vi "Rotation stage shgv6.vi"() -> ()   [LabVIEW 2020]
doc: "Shows how to move a motor to an absolute position."
uses:
  <vilib>/Utility/error.llb/DialogType.ctl
  <vilib>/DAQmx/read.llb/DAQmx Read (Analog 1D Wfm NChan 1Samp).vi
  <vilib>/DAQmx/read.llb/DAQmx Read (Counter 1D U32 1Chan NSamp).vi
  <vilib>/DAQmx/create/channels.llb/DAQmx Create Channel (CI-Period).vi
  <vilib>/DAQmx/create/channels.llb/DAQmx Create Channel (CO-Pulse Generation-Frequency).vi
  <vilib>/DAQmx/configure/timing.llb/DAQmx Timing (Implicit).vi
  <vilib>/DAQmx/miscellaneous.llb/DAQmx Fill In Error Info.vi
  <vilib>/DAQmx/create/channels.llb/DAQmx Create Channel (AI-Current-Basic).vi
  <vilib>/DAQmx/configure/timing.llb/DAQmx Timing (Sample Clock).vi
  <resource>/objmgr/daqmx.rc
panel:
  in  "stop":bool
  in  "MG17Motor":refnum<k7>(container)
  in  "Home":bool
  in  "Move Relative":bool
  in  "Rel Move Size":dbl=1.0 min=-10.0 max=10.0 format="%.2f"
  in  "Set Rel Move Size":bool
  in  "Stop":bool
  out "Actual Sample Rate":dbl=1000.0 format="%0.2f"
  out "Reference Channel":waveform(dbl)[](graph)
  out "Consumer Iteration 3":i32=1109257
  out "Producer Iteration 3":i32=1109256
  out "error out 3":errorcluster
  out "Loop Time (ms) 3":u32=10
  in  "Duty Cycle":dbl=0.5 format="%.6f"
  out "Input.BufSize":u32=1000000 format="%.0p"
  out "PC-PMT":u32[](graph)
  out "Consumer Iteration 2":i32=1109257
  in  "number of samples per channel 2":i32=5000
  out "Producer Iteration 2":i32=1109256
  out "error out 2":errorcluster
  out "Loop Time (ms) 2":u32=10
  in  "dwell time (ms)":dbl=1.0 format="%.6f"
  in  "Photon Input (PFI)":tag="/Dev1/PFI0"
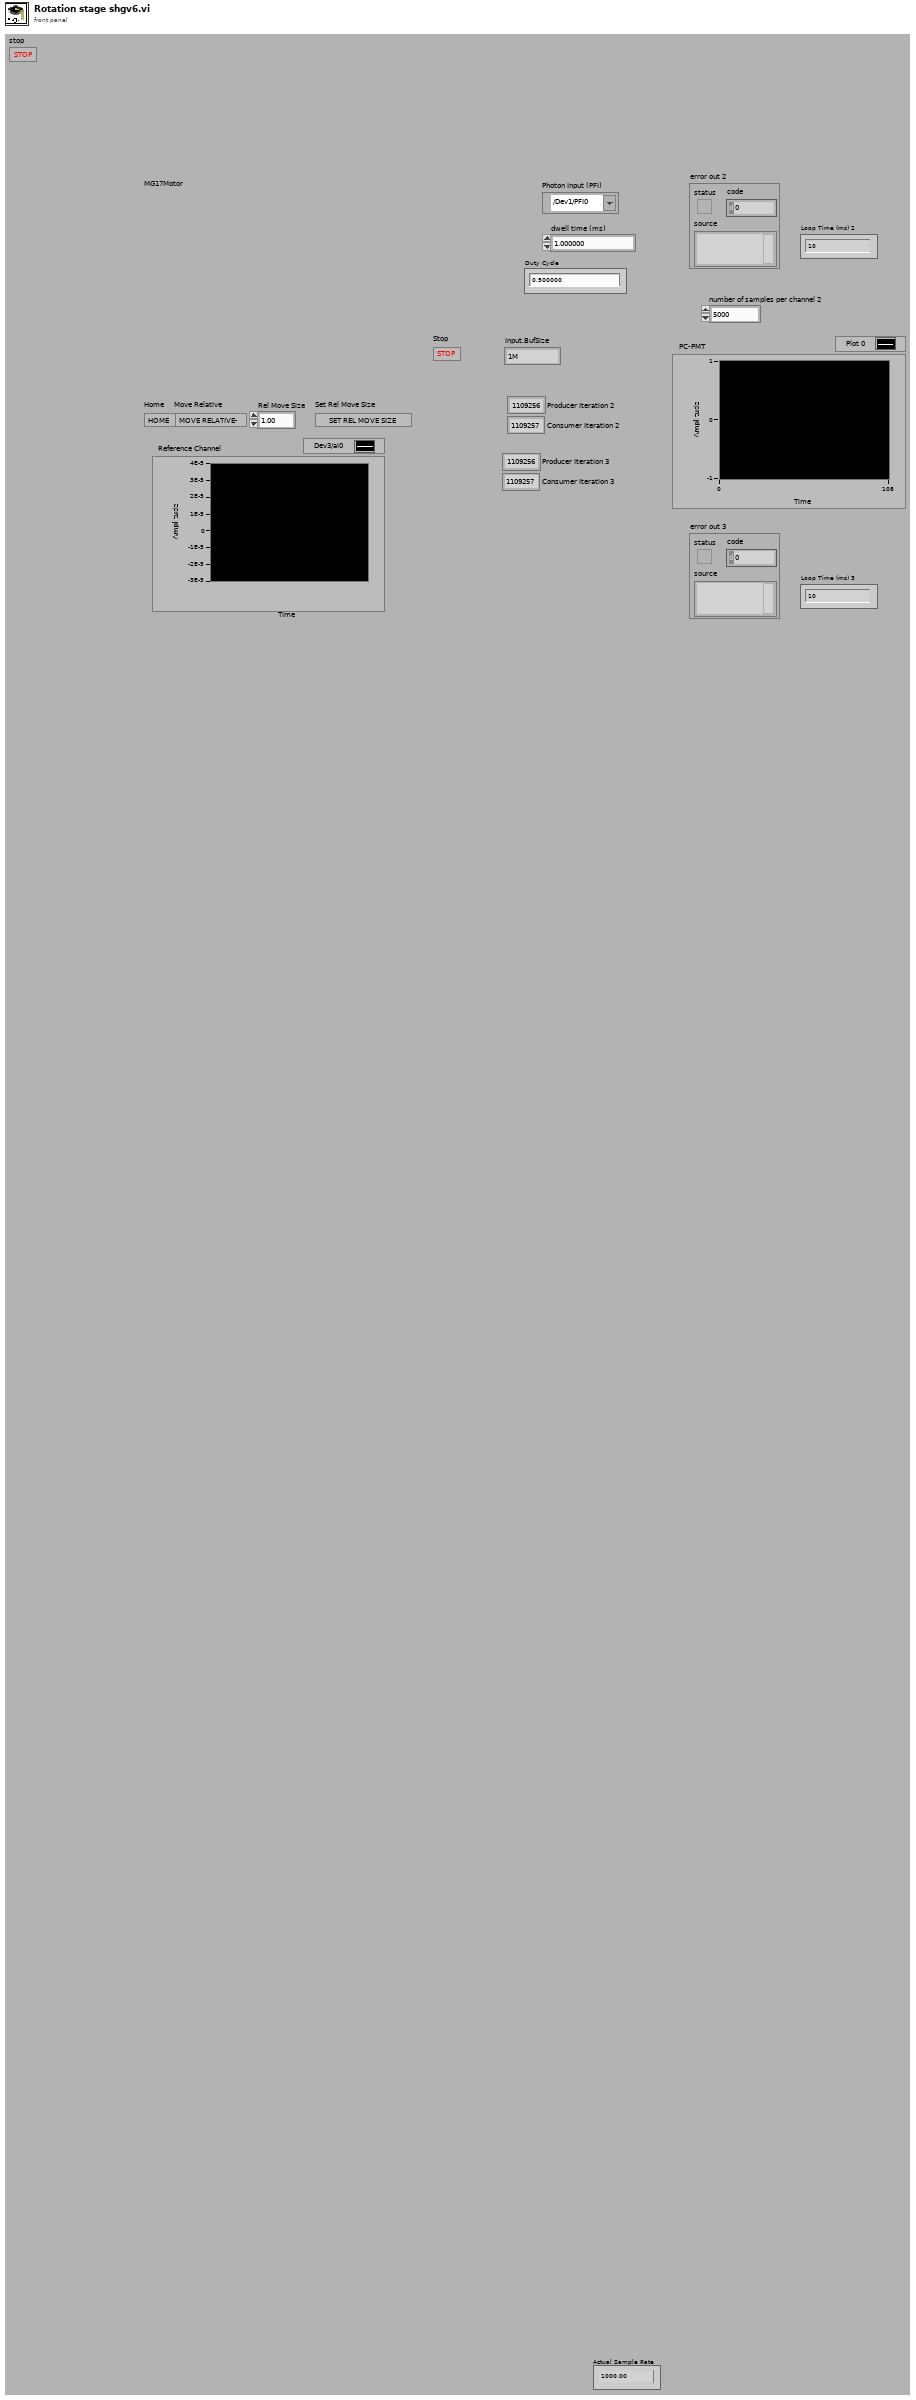
[diagram p1: front panel]
types:
  T1 = enum16{"open", "open or create", "create or replace", "create", "open (read-only)"}
  T2 = typedef "DialogType.ctl" = u16
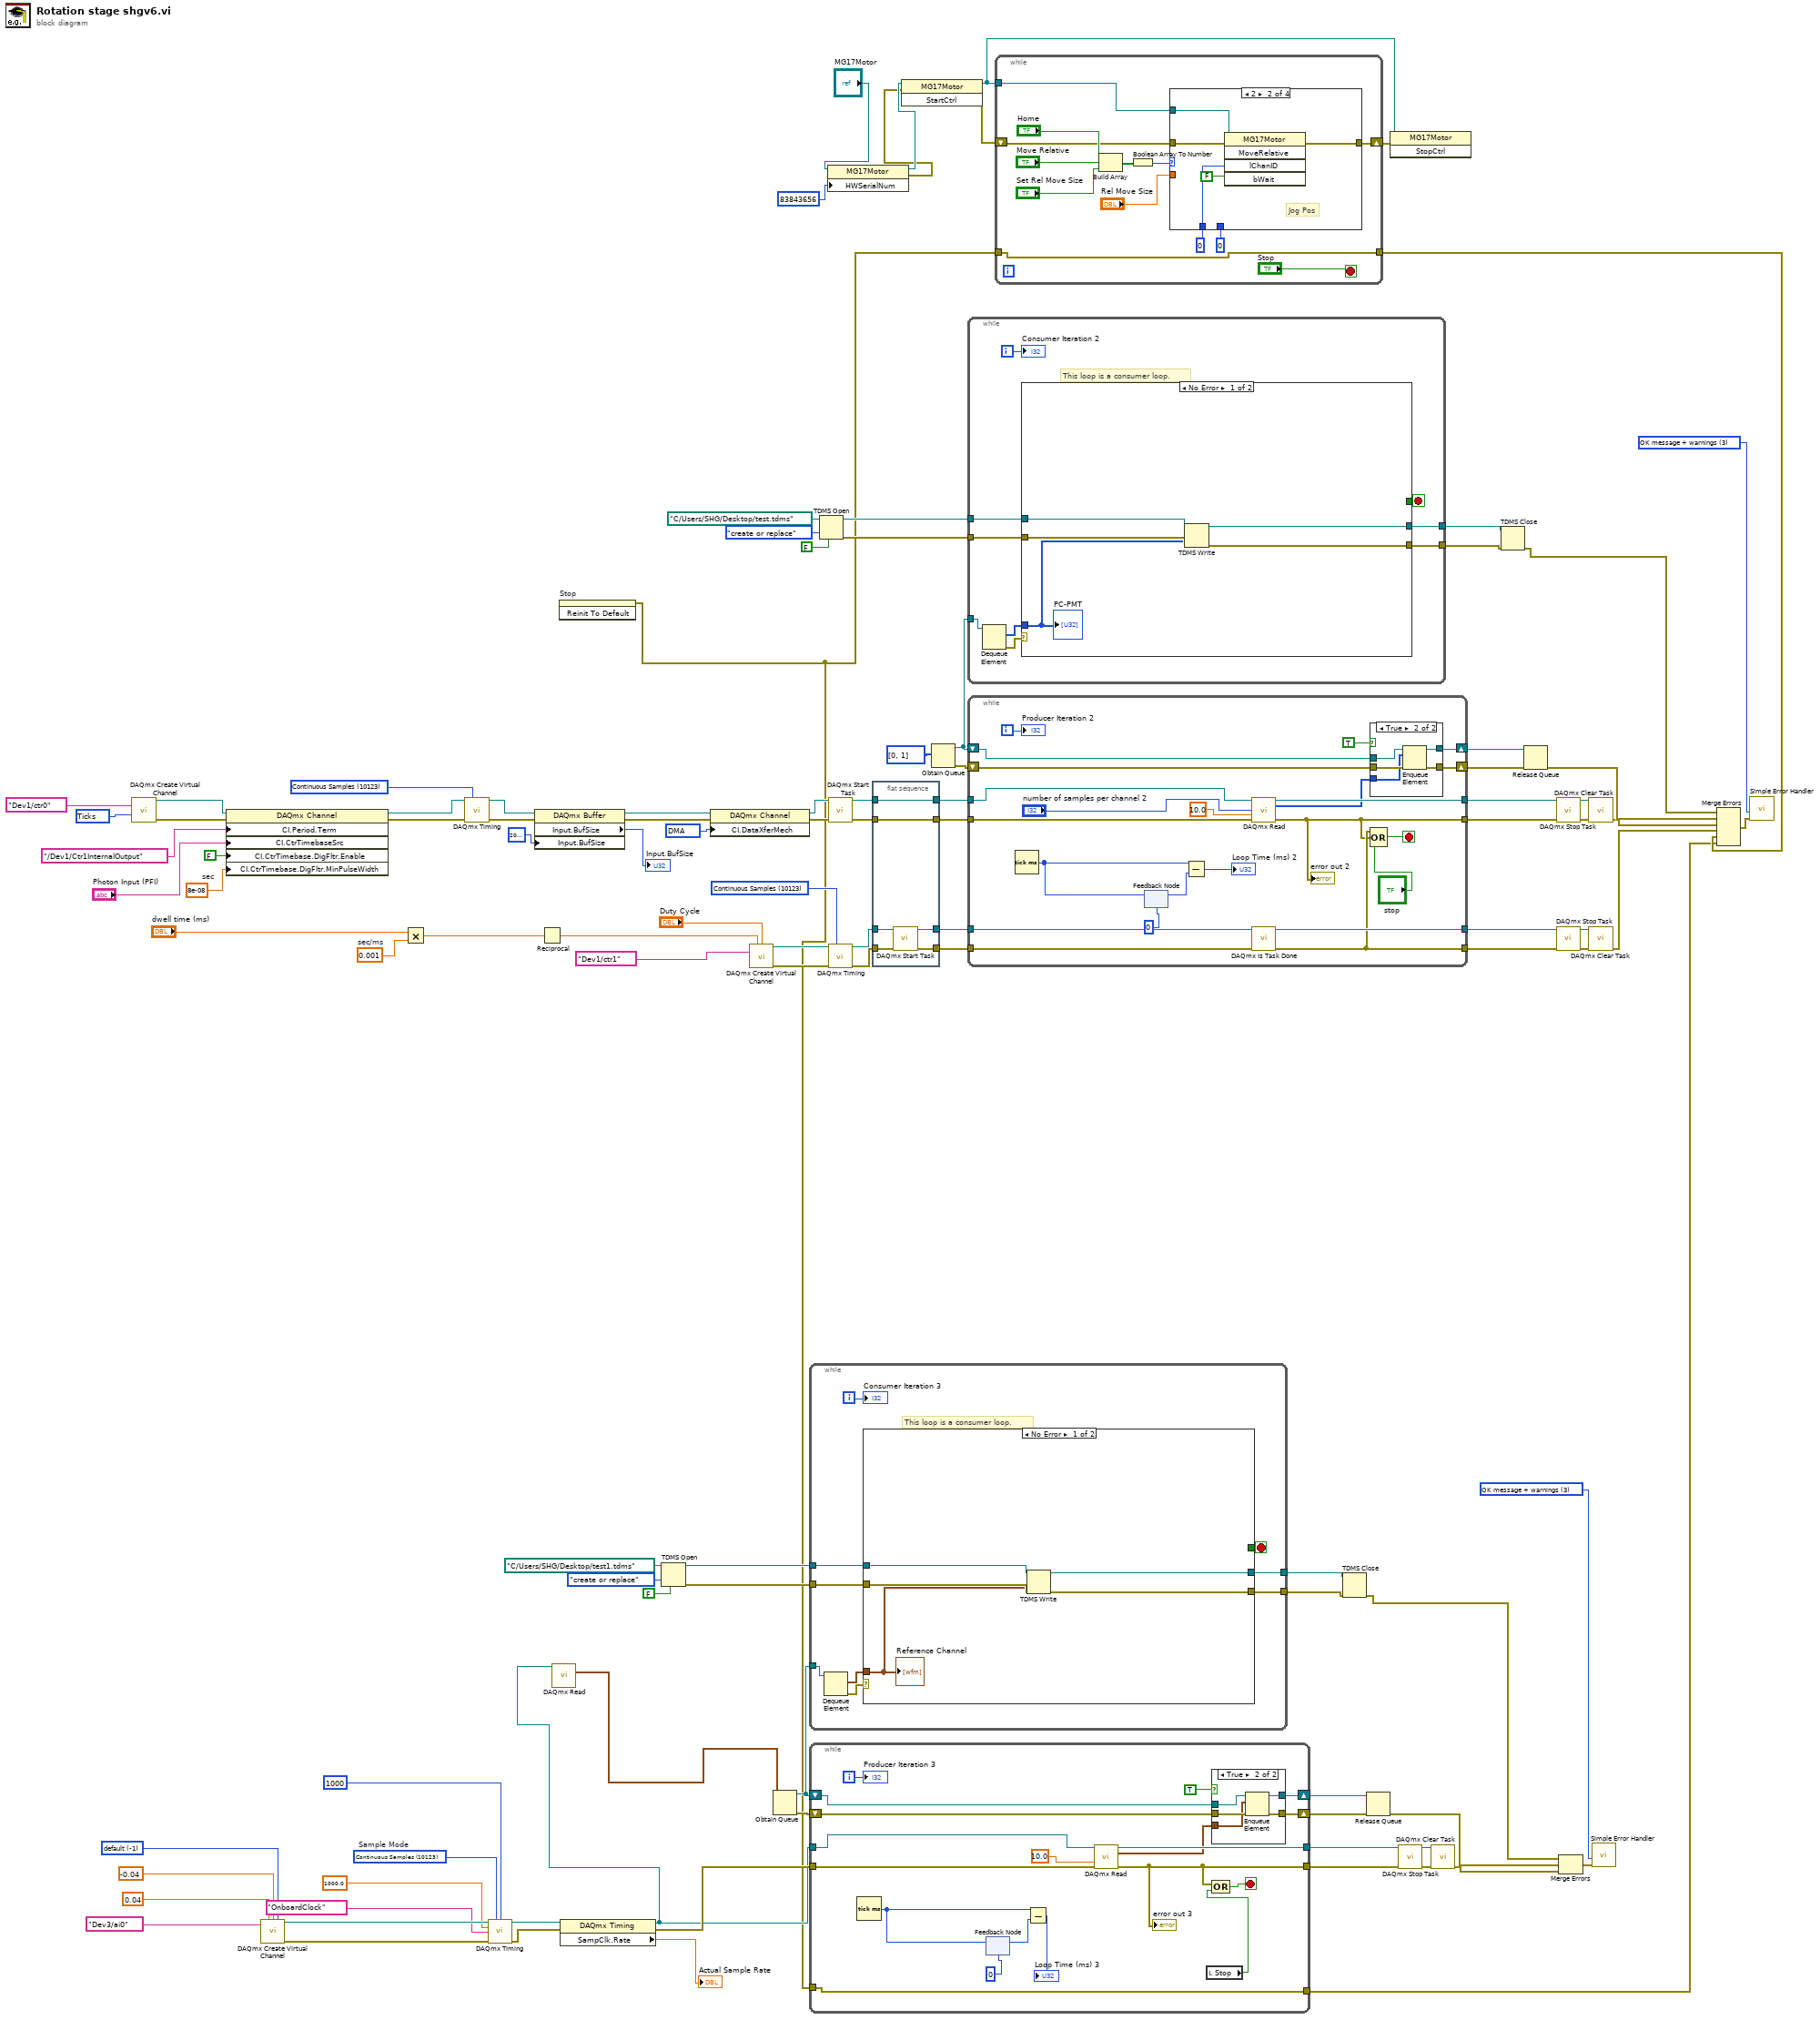
[diagram p0: block diagram]
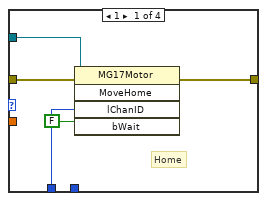
[diagram p2: hidden frame]
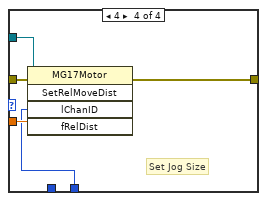
[diagram p4: hidden frame]
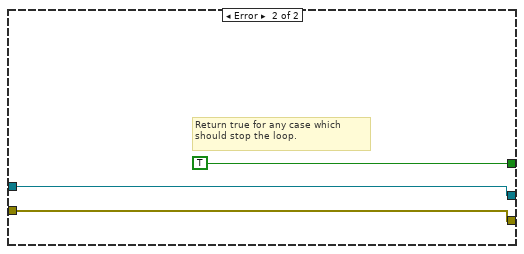
[diagram p5: hidden frame]
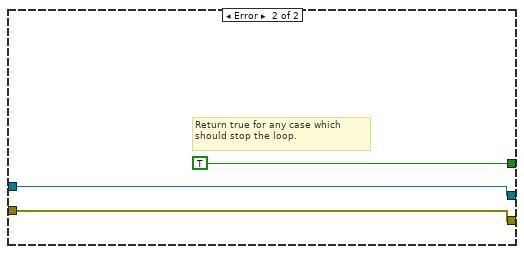
[diagram p7: hidden frame]
diagram:
  w16 = -1 items=["default"=-1, "RSE"=10083, "NRSE"=10078, "Differential"=10106, "Pseudodifferential"=12529] ("Terminal Configuration")
  w24 = 10123 items=["Finite Samples"=10178, "Continuous Samples"=10123, "Hardware Timed Single Point"=12522]  # Sample Mode
  w34 = T2 3 items=["no dialog", "OK message", "continue or stop message", "OK message + warnings", "continue/stop + warnings"] ("type of dialog (OK msg:1)")
  w55 = T2 3 items=["no dialog", "OK message", "continue or stop message", "OK message + warnings", "continue/stop + warnings"] ("type of dialog (OK msg:1)")
  w60 = 8e-08  # sec
  w71 = 10054 items=["DMA"=10054, "Interrupts"=10204, "Programmed I/O"=10264, "USB Bulk"=12590] ("CI.DataXferMech")
  w91 = 0.001  # sec/ms
  w101 = 10304 items=["Seconds"=10364, "Ticks"=10304, "From Custom Scale"=10065] ("units")
  w102 = 10123 items=["Finite Samples"=10178, "Continuous Samples"=10123, "Hardware Timed Single Point"=12522] ("sample mode")
  w103 = 10123 items=["Finite Samples"=10178, "Continuous Samples"=10123, "Hardware Timed Single Point"=12522] ("sample mode")
  n1 = call-poly <vilib>:"DAQmx Create Virtual Channel.vi"("counter"=tag "Dev1/ctr0", "units"=w101) -> ("task out"=w98:refnum<k21>, "error out"=w97:errorcluster)  [unwired: 12 in]
  n2 = property class="DAQmx Channel"(reference=w98, error in=w97, "CI.Period.Term"=tag "/Dev1/Ctr1InternalOutput", "CI.CtrTimebaseSrc"="Photon Input (PFI)", "CI.CtrTimebase.DigFltr.Enable"=FALSE, "CI.CtrTimebase.DigFltr.MinPulseWidth"=w60) -> (reference out=w96:refnum<k21>, error out=w95:errorcluster)
  n3 = call-poly <vilib>:"DAQmx Create Virtual Channel.vi"("maximum value"=0.04 ("Max Voltage"), "minimum value"=-0.04 ("Min Voltage"), "input terminal configuration"=w16, "physical channels"=tag "Dev3/ai0" ("Physical Channel")) -> ("task out"=w22:refnum<k21>, "error out"=w23:errorcluster)  [unwired: 10 in]
  n4 = Multiply(x="dwell time (ms)", y=w91) -> (x*y=w90:dbl)
  n5 = call-poly <vilib>:"DAQmx Timing.vi"("task/channels in"=w96, "sample mode"=w102, "error in"=w95) -> ("task out"=w66:refnum<k21>, "error out"=w65:errorcluster)  [unwired: 11 in]
  n6 = call-poly <vilib>:"DAQmx Timing.vi"("task/channels in"=w22, "sample mode"=w24, "samples per channel"=1000 ("Number of Samples"), "rate"=1000.0 ("Sample Rate"), "source"=tag "OnboardClock" ("Sample Clock Source"), "error in"=w23) -> ("task out"=w26:refnum<k21>, "error out"=w25:errorcluster)  [unwired: 8 in]
  n7 = property class="DAQmx Buffer"(reference=w66, error in=w65, "Input.BufSize"=u32 2000000 ("samples per channel")) -> (reference out=w70:refnum<k21>, error out=w68:errorcluster, "Input.BufSize"=→"Input.BufSize":u32)
  n8 = Reciprocal(x=w90) -> (1/x=w89:dbl)
  n9 = invoke on="Stop" class="Bool (strict)" method="Reinit To Default"() -> (error out=w3:errorcluster)  [unwired: 3 in, 2 out]
  n10 = property class="DAQmx Timing"(reference=w26, error in=w25) -> (reference out=w11:refnum<k21>, error out=w20:errorcluster, "SampClk.Rate"=→"Actual Sample Rate":dbl)
  n11 = call-poly <vilib>:"DAQmx Read.vi"("task/channels in"=w11) -> ("data"=w12:waveform(dbl)[])  [unwired: 12 in, 2 out]
  n12 = TDMS Open(6:FALSE ("disable buffering? (T)"), 10:T1."create or replace" ("operation (0:open)"), 11:path "C:/Users/SHG/Desktop/test1.tdms" ("file path")) -> (0:w36:errorcluster, 3:w38:refnum<k34>)  [unwired: 4 in]
  n13 = property class="DAQmx Channel"(reference=w70, error in=w68, "CI.DataXferMech"=w71) -> (reference out=w64:refnum<k21>, error out=w63:errorcluster)
  n14 = call-poly <vilib>:"DAQmx Create Virtual Channel.vi"("frequency"=w89, "duty cycle"="Duty Cycle", "counter"=tag "Dev1/ctr1") -> ("task out"=w108:refnum<k21>, "error out"=w109:errorcluster)  [unwired: 11 in]
  n15 = Obtain Queue(element data type=w12) -> (queue out=w46:refnum<queue>, error out=w45:errorcluster)  [unwired: 4 in, 1 out]
  n16 = while {
    tunnel: w46 -> [w118]
    tunnel: w38 -> [w113]
    tunnel: [w112] -> w37
    tunnel: w36 -> [w111]
    tunnel: [w110] -> w35
    i -> [w114]
    stop <- w115 stop-if-true
    # "This loop is a consumer loop."
    n17 = Dequeue Element(queue=w118) -> (element=w116:waveform(dbl)[], error out=w117:errorcluster)  [unwired: 2 in, 2 out]
    n18 = case shown="No Error" w117 {
      tunnel: w116 -> [w119 _]
      tunnel: [_ TRUE] -> w115
      tunnel: w113 -> [w123 w125]
      tunnel: [w122 w125] -> w112
      tunnel: w111 -> [w121 w124]
      tunnel: [w120 w124] -> w110
      frame No Error {
        n19 = TDMS Write(0:w123, 9:w119, 11:w121) -> (4:w122:refnum<k34>, 15:w120:errorcluster)  [unwired: 3 in, 2 out]
        "Reference Channel" <- w119
      }
      frame Error {
        # "Return true for any case which should stop the loop."
      }
    }
    "Consumer Iteration 3" <- w114
  }
  n20 = while {
    shift-right: [w135] -> w43
    shift-left: w45 -> [w143]
    shift-right: [w144] -> w44
    shift-left: w46 -> [w145]
    tunnel: [w141] -> w40
    tunnel: [w134] -> w39
    tunnel: w20 -> [w140]
    tunnel: w11 -> [w139]
    tunnel: w3 -> [w127]
    tunnel: [w127] -> w1
    i -> [w136]
    stop <- w133 stop-if-true
    n21 = Tick Count (ms)() -> (millisecond timer value=w132:u32)
    n22 = feedback #1(u32 0 ("millisecond timer value")) -> (w131:u32)
    n23 = feedback-in #1(w132) -> ()
    n24 = Subtract(x=w132, y=w131) -> (x-y=→"Loop Time (ms) 3":u32)
    n25 = call-poly <vilib>:"DAQmx Read.vi"("task/channels in"=w139, "timeout"=10.0, "error in"=w140) -> ("task out"=w141:refnum<k21>, "data"=w138:waveform(dbl)[], "error out"=w134:errorcluster)  [unwired: 10 in]
    "error out 3" <- w134
    n26 = local read "Stop"() -> (w128:bool)
    n27 = case shown="True" TRUE ("Case Constant\n(See Context Help)") {
      tunnel: w145 -> [w147 w152]
      tunnel: [w147 w151] -> w144
      tunnel: w143 -> [w146 w150]
      tunnel: [w146 w149] -> w135
      tunnel: w138 -> [_ w148]
      frame False {
      }
      frame True {
        n28 = Enqueue Element(queue=w152, element=w148, error in (no error)=w150) -> (queue out=w151:refnum<queue>, error out=w149:errorcluster)  [unwired: 1 in, 1 out]
      }
    }
    n29 = Compound Arithmetic op=OR(w134, w128) -> (w133:bool)
    "Producer Iteration 3" <- w136
  }
  n30 = TDMS Open(6:FALSE ("disable buffering? (T)"), 10:T1."create or replace" ("operation (0:open)"), 11:path "C:/Users/SHG/Desktop/test.tdms" ("file path")) -> (0:w57:errorcluster, 3:w59:refnum<k34>)  [unwired: 4 in]
  n31 = property class="MG17Motor"(reference="MG17Motor", "HWSerialNum"=83843656) -> (reference out=w5:refnum<k7>, error out=w4:errorcluster)  [unwired: 1 in]
  n32 = call <vilib>:"DAQmx Start Task.vi"("task/channels in"=w64, "error in"=w63) -> ("task out"=w88:refnum<k21>, "error out"=w87:errorcluster)  [unwired: 12 in]
  n33 = call-poly <vilib>:"DAQmx Timing.vi"("task/channels in"=w108, "sample mode"=w103, "error in"=w109) -> ("task out"=w107:refnum<k21>, "error out"=w106:errorcluster)  [unwired: 11 in]
  n34 = flat-sequence {
    tunnel: w107 -> [w158]
    tunnel: w106 -> [w157]
    tunnel: [w156] -> w74
    tunnel: [w155] -> w75
    tunnel: w88 -> [w153]
    tunnel: w87 -> [w154]
    tunnel: [w154] -> w77
    tunnel: [w153] -> w76
    frame #0 {
      n35 = call <vilib>:"DAQmx Start Task.vi"("task/channels in"=w158, "error in"=w157) -> ("task out"=w155:refnum<k21>, "error out"=w156:errorcluster)  [unwired: 12 in]
    }
  }
  n36 = invoke class="MG17Motor" method="StartCtrl"(reference=w5, error in=w4) -> (reference out=w10:refnum<k7>, error out=w9:errorcluster)  [unwired: 1 in, 1 out]
  n37 = Obtain Queue(element data type=u32[] [0, 1] ("data")) -> (queue out=w86:refnum<queue>, error out=w85:errorcluster)  [unwired: 4 in, 1 out]
  n38 = while {
    tunnel: w86 -> [w167]
    tunnel: w59 -> [w162]
    tunnel: [w161] -> w58
    tunnel: w57 -> [w160]
    tunnel: [w159] -> w56
    i -> [w163]
    stop <- w164 stop-if-true
    # "This loop is a consumer loop."
    n39 = Dequeue Element(queue=w167) -> (element=w165:u32[], error out=w166:errorcluster)  [unwired: 2 in, 2 out]
    n40 = case shown="No Error" w166 {
      tunnel: w165 -> [w168 _]
      tunnel: [_ TRUE] -> w164
      tunnel: w162 -> [w172 w174]
      tunnel: [w171 w174] -> w161
      tunnel: w160 -> [w170 w173]
      tunnel: [w169 w173] -> w159
      frame No Error {
        n41 = TDMS Write(0:w172, 9:w168, 11:w170) -> (4:w171:refnum<k34>, 15:w169:errorcluster)  [unwired: 3 in, 2 out]
        "PC-PMT" <- w168
      }
      frame Error {
        # "Return true for any case which should stop the loop."
      }
    }
    "Consumer Iteration 2" <- w163
  }
  n42 = while {
    shift-right: [w187] -> w83
    shift-left: w85 -> [w196]
    shift-right: [w197] -> w84
    shift-left: w86 -> [w198]
    tunnel: [w194] -> w80
    tunnel: [w182] -> w79
    tunnel: w77 -> [w193]
    tunnel: w76 -> [w192]
    tunnel: w75 -> [w186]
    tunnel: w74 -> [w185]
    tunnel: [w184] -> w73
    tunnel: [w183] -> w72
    i -> [w188]
    stop <- w181 stop-if-true
    n43 = Tick Count (ms)() -> (millisecond timer value=w180:u32)
    n44 = feedback #2(u32 0 ("millisecond timer value")) -> (w179:u32)
    n45 = feedback-in #2(w180) -> ()
    n46 = Subtract(x=w180, y=w179) -> (x-y=→"Loop Time (ms) 2":u32)
    n47 = call-poly <vilib>:"DAQmx Read.vi"("task/channels in"=w192, "number of samples per channel"="number of samples per channel 2", "timeout"=10.0, "error in"=w193) -> ("task out"=w194:refnum<k21>, "data"=w191:u32[], "error out"=w182:errorcluster)  [unwired: 9 in]
    "error out 2" <- w182
    n48 = call <vilib>:"DAQmx Is Task Done.vi"("task/channels in"=w186, "error in"=w185) -> ("task out"=w184:refnum<k21>, "error out"=w183:errorcluster)  [unwired: 11 in, 1 out]
    n49 = case shown="True" TRUE ("Case Constant\n(See Context Help)") {
      tunnel: w198 -> [w200 w205]
      tunnel: [w200 w204] -> w197
      tunnel: w196 -> [w199 w203]
      tunnel: [w199 w202] -> w187
      tunnel: w191 -> [_ w201]
      frame False {
      }
      frame True {
        n50 = Enqueue Element(queue=w205, element=w201, error in (no error)=w203) -> (queue out=w204:refnum<queue>, error out=w202:errorcluster)  [unwired: 1 in, 1 out]
      }
    }
    n51 = Compound Arithmetic op=OR(w183, w182, "stop") -> (w181:bool)
    "Producer Iteration 2" <- w188
  }
  n52 = while {
    shift-left: w9 -> [w211]
    shift-right: [w212] -> w8
    tunnel: w10 -> [w216]
    tunnel: w3 -> [w206]
    tunnel: [w206] -> w2
    stop <- "Stop" stop-if-true
    n53 = Build Array("Home", "Move Relative", "Set Rel Move Size") -> (w209:bool[])
    n54 = Boolean Array To Number(Boolean array=w209) -> (number=w210:u32)
    n55 = case shown="2" w210 {
      tunnel: w216 -> [w223 w228 _ w234]
      tunnel: 0 ("lChanID") -> [w222 w227 _ _]
      tunnel: "Rel Move Size" -> [_ _ _ w233]
      tunnel: [w221 w226 w229 w231] -> w212
      tunnel: w211 -> [w220 w224 w229 w230]
      tunnel: 0 ("lChanID") -> [_ _ _ w232]
      frame 1 {
        # "Home"
        n56 = invoke class="MG17Motor" method="MoveHome"(reference=w223, error in=w220, "lChanID"=w222, "bWait"=FALSE) -> (error out=w221:errorcluster)  [unwired: 1 in, 4 out]
      }
      frame 2 {
        # "Jog Pos"
        n57 = invoke class="MG17Motor" method="MoveRelative"(reference=w228, error in=w224, "lChanID"=w227, "bWait"=FALSE) -> (error out=w226:errorcluster)  [unwired: 1 in, 4 out]
      }
      frame Default {
      }
      frame 4 {
        # "Set Jog Size"
        n58 = invoke class="MG17Motor" method="SetRelMoveDist"(reference=w234, error in=w230, "lChanID"=w232, "fRelDist"=w233) -> (error out=w231:errorcluster)  [unwired: 1 in, 4 out]
      }
    }
  }
  n59 = TDMS Close(8:w35, 11:w37) -> (0:w30:errorcluster)  [unwired: 1 out]
  n60 = Release Queue(queue=w44, error in (no error)=w43) -> (error out=w29:errorcluster)  [unwired: 1 in, 2 out]
  n61 = invoke class="MG17Motor" method="StopCtrl"(reference=w10, error in=w8) -> ()  [unwired: 1 in, 3 out]
  n62 = call <vilib>:"DAQmx Stop Task.vi"("task/channels in"=w40, "error in"=w39) -> ("task out"=w41:refnum<k21>, "error out"=w42:errorcluster)  [unwired: 12 in]
  n63 = call <vilib>:"DAQmx Clear Task.vi"("task in"=w41, "error in"=w42) -> ("error out"=w28:errorcluster)  [unwired: 13 in]
  n64 = TDMS Close(8:w56, 11:w58) -> (0:w51:errorcluster)  [unwired: 1 out]
  n65 = Release Queue(queue=w84, error in (no error)=w83) -> (error out=w50:errorcluster)  [unwired: 1 in, 2 out]
  n66 = call <vilib>:"DAQmx Stop Task.vi"("task/channels in"=w80, "error in"=w79) -> ("task out"=w81:refnum<k21>, "error out"=w82:errorcluster)  [unwired: 12 in]
  n67 = call <vilib>:"DAQmx Stop Task.vi"("task/channels in"=w73, "error in"=w72) -> ("task out"=w105:refnum<k21>, "error out"=w104:errorcluster)  [unwired: 12 in]
  n68 = Merge Errors(w30, w29, w28) -> (w33:errorcluster)
  n69 = call <vilib>:"DAQmx Clear Task.vi"("task in"=w81, "error in"=w82) -> ("error out"=w49:errorcluster)  [unwired: 13 in]
  n70 = call <vilib>:"DAQmx Clear Task.vi"("task in"=w105, "error in"=w104) -> ("error out"=w48:errorcluster)  [unwired: 13 in]
  n71 = call <vilib>:"Simple Error Handler.vi"("type of dialog (OK msg:1)"=w34, "error in (no error)"=w33) -> ()  [unwired: 3 in, 5 out]
  n72 = Merge Errors(w51, w50, w49, w48, w2, w1) -> (w54:errorcluster)
  n73 = call <vilib>:"Simple Error Handler.vi"("type of dialog (OK msg:1)"=w55, "error in (no error)"=w54) -> ()  [unwired: 3 in, 5 out]
